vi "svl_Build Scaling Array for Frequency Domain Integration.vi"(9 "integration type":T2(ring), 10 "spectrum type":T1=enum."Power [Magnitude^2]", 11 "frequency array [Hz]":dbl[](array[numeric]) format="%.2f") -> (2 "dB multiplier":dbl format="%.2f", 3 "scaling array":dbl[](array[numeric]) format="%.2f")   [LabVIEW 2017, in "SoundVib_Integration.lvlib"]
uses:
  <vilib>/addons/Sound and Vibration/svt_Integration/SoundVib_Integration.lvlib
  <vilib>/addons/_NISVFA/_Shared subVIs/Controls/svc_Spectrum Type.ctl
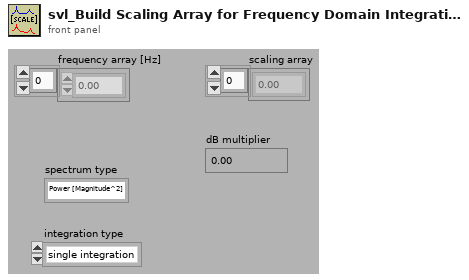
[diagram p1: front panel]
types:
  T1 = typedef "svc_Spectrum Type.ctl" = enum16{"FFT Spectrum [complex]", "Amplitude [Magnitude]", "Power [Magnitude^2]", "Cross Spectrum [complex]", "Frequency Response [Complex]"}
  T2 = enum16{"single integration", "double integration"}
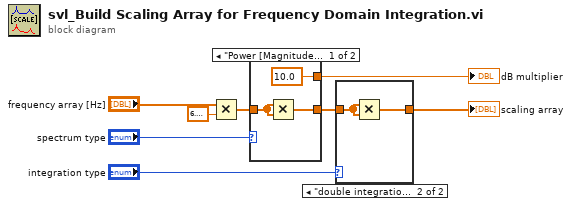
[diagram p0: block diagram]
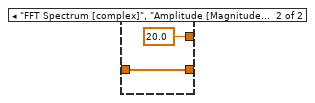
[diagram p2: hidden frame]
diagram:
  n1 = Multiply(x="frequency array [Hz]", y=6.283185307179586) -> (x*y=w2:dbl[])
  n2 = case shown="\"Power [Magnitude^2]\", \"Cross Spectrum [complex]\", Default" "spectrum type" {
    tunnel: w2 -> [w11 w13]
    tunnel: [w10 w13] -> w1
    tunnel: [10.0 20.0] -> w5
    frame "Power [Magnitude^2]", "Cross Spectrum [complex]", Default {
      n3 = Multiply(x=w11, y=w11) -> (x*y=w10:dbl[])
    }
    frame "FFT Spectrum [complex]", "Amplitude [Magnitude]", "Frequency Response [Complex]" {
    }
  }
  "dB multiplier" <- w5
  n4 = case shown="\"double integration\"" "integration type" {
    tunnel: w1 -> [w14 w16]
    tunnel: [w14 w15] -> w6
    frame "single integration", Default {
    }
    frame "double integration" {
      n5 = Multiply(x=w16, y=w16) -> (x*y=w15:dbl[])
    }
  }
  "scaling array" <- w6
